vi "TMP007 Init.vi"(7 "I2C Channel":u8=1, 8 "error in (no error)":errorcluster, 9 "Samples to Average":u16(ring) items=["1 sample, .26s conversion"=0, "2 samples, .51s conversion"=512, "4 samples, 1.01s conversion"=1024, "8 samples, 2.01s conversion"=1536, "16 samples, 4.01s conversion"=2048], 10 "I2C Slave Address":u8=64 format="%.0x", 11 "LINX Resource in":T2) -> (0 "error out":errorcluster, 2 "Thermopile Setting":T1={"Samples to Average"=0, "I2C Slave Address"=64, "I2C Channel"=1, "Online"=FALSE} {"I2C Slave Address" format="%.0x"; "Samples to Average" items=["1 sample, .26s conversion"=0, "2 samples, .51s conversion"=512, "4 samples, 1.01s conversion"=1024, "8 samples, 2.01s conversion"=1536, "16 samples, 4.01s conversion"=2048]}, 3 "LINX Resource out":T2)   [LabVIEW 2014]
uses:
  <vilib>/MakerHub/LINX/Private/Type Defs/LINX Ref.ctl
  <vilib>/MakerHub/LINX/Private/Type Defs/Platform.ctl
  <vilib>/MakerHub/LINX/Private/Type Defs/Interface.ctl
  <vilib>/MakerHub/LINX/Private/Device/Type Defs/LINX Device Config.ctl
  <vilib>/MakerHub/LINX/Private/Device/Type Defs/TCP Config.ctl
  <vilib>/MakerHub/LINX/Private/Device/Type Defs/Channels.ctl
  <vilib>/MakerHub/LINX/Private/Local IO/LinxI2cWrite.vi
  <vilib>/MakerHub/LINX/Public/Utilities/Check Channel.vi
  <vilib>/myRIO/Instrument Drivers/Onboard IO/I2C/vis/Write.vi
  <vilib>/MakerHub/LINX/Private/Utilties/Generate Error.vi
  <vilib>/MakerHub/LINX/Private/Utilties/Channel FGVs/I2C Channels.vi
  <vilib>/Utility/error.llb/Error Cluster From Error Code.vi
  <vilib>/myRIO/Common/Instrument Driver Framework/myRIO v1.0/I2C/vis/myRIO v1.0 Write I2C.vi
  <vilib>/MakerHub/LINX/LMH-LINX.lvlib
  <vilib>/MakerHub/LINX/Private/Device/Device.lvlib
panel:
  # "Each sample takes .25s to convert\nThere are some other conversion modes that include idle times, but I didn't include those modes"
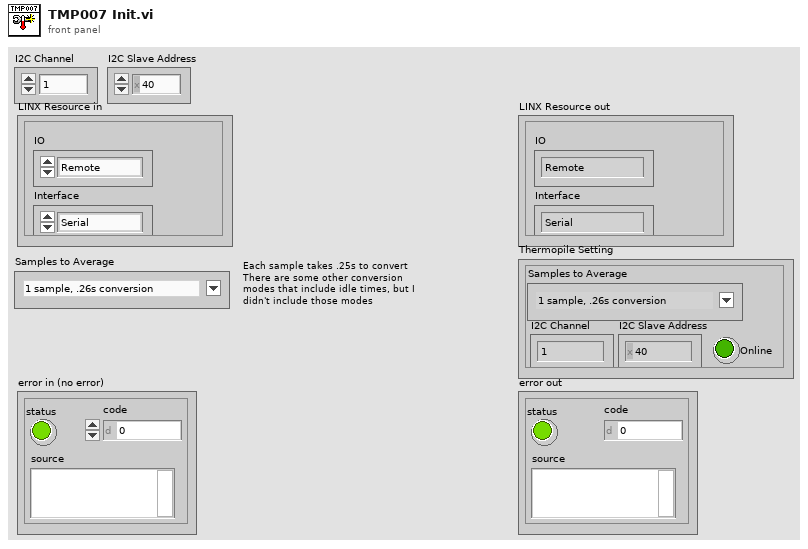
[diagram p1: front panel]
types:
  T1 = cluster{"Samples to Average":u16, "I2C Slave Address":u8, "I2C Channel":u8, "Online":bool}
  T2 = typedef "LMH-LINX.lvlib/LINX Ref.ctl" = cluster{"IO":T3, "Interface":T4, "LINX Device Config":T5}
  T3 = typedef "LMH-LINX.lvlib/Platform.ctl" = enum16{"Remote", "Local"}
  T4 = typedef "LMH-LINX.lvlib/Interface.ctl" = enum16{"Serial", "TCP"}
  T5 = typedef "LMH-LINX.lvlib/Device.lvlib/LINX Device Config.ctl" = cluster{"Interface":T4, "COM Port":refnum<visa-resource-name>, "TCP Configuration":T6, "Device Family":u8, "Device ID":u8, "Device Name":string, "TCP Ref":refnum<k5>, "Channels":T7}
  T6 = typedef "LMH-LINX.lvlib/Device.lvlib/TCP Config.ctl" = cluster{"IP Address":string, "Port":u16}
  T7 = typedef "LMH-LINX.lvlib/Channels.ctl" = cluster{"DI":u8[], "DO":u8[], "AI":u8[], "AO":u8[], "PWM":u8[], "QE":u8[], "UART":u8[], "I2C 2":u8[], "SPI":u8[], "CAN":u8[], "Servo":u8[], "AI Ref (V)":dbl, "AI Resolution (Bits)":u8, "AO Ref (V)":dbl, "AO Resolution (Bits)":u8}
  T8 = cluster{"Samples to Average":u16, "I2C Slave Address":u8, "I2C Channel":u8, bool}
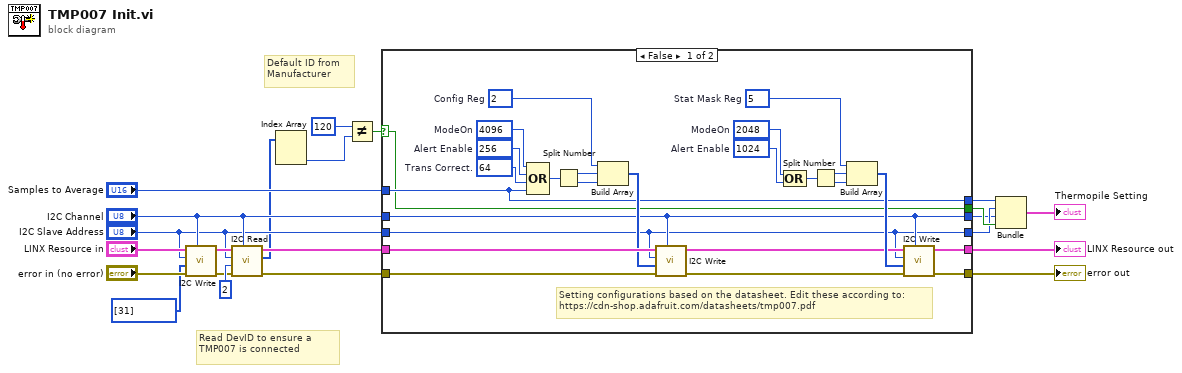
[diagram p0: block diagram]
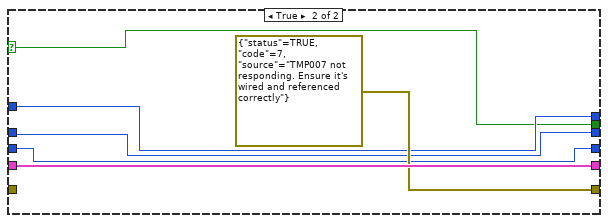
[diagram p2: hidden frame]
diagram:
  # "Default ID from Manufacturer"
  # "Read DevID to ensure a TMP007 is connected"
  n1 = call <vilib>:"I2C Write.vi"("I2C Channel"="I2C Channel", "Error In"="error in (no error)", "Data"=u8[] [31], "I2C Slave Address (0)"="I2C Slave Address", "LINX Resource"="LINX Resource in") -> ("Error Out"=w15:errorcluster, "LINX Resource"=w14:T2)  [unwired: 5 in]
  n2 = call <vilib>:"I2C Read.vi"("I2C Channel"="I2C Channel", "Error In"=w15, "Bytes To Read"=u8 2, "I2C Slave Address (0)"="I2C Slave Address", "LINX Resource"=w14) -> ("Error Out"=w18:errorcluster, "Data"=w8:u8[], "LINX Resource"=w19:T2)  [unwired: 4 in]
  n3 = Index Array(array=w8) -> (element #2=w6:u8)  [unwired: 2 in, 1 out]
  n4 = Not Equal?(x=u8 120, y=w6) -> (x != y?=w12:bool)
  n5 = case shown="False" w12 {
    selector: w12 -> [w25 w50]
    tunnel: w19 -> [w47 w53]
    tunnel: [w28 w53] -> w21
    tunnel: w18 -> [w46 _]
    tunnel: [w27 errorcluster {"status"=TRUE, "code"=7, "source"="TMP007 not responding. Ensure it's wired and referenced correctly"} ("error constant")] -> w20
    tunnel: "Samples to Average" -> [w26 w51]
    tunnel: "I2C Channel" -> [w24 w49]
    tunnel: "I2C Slave Address" -> [w23 w48]
    tunnel: [w26 w51] -> w5
    tunnel: [w25 w50] -> w4
    tunnel: [w24 w49] -> w1
    tunnel: [w23 w48] -> w2
    frame False {
      w37 = u8 5  # Stat Mask Reg
      w32 = u16 1024  # Alert Enable
      w33 = u16 2048  # ModeOn
      w39 = u8 2  # Config Reg
      w45 = u16 64  # Trans Correct.
      w44 = u16 256  # Alert Enable
      w43 = u16 4096  # ModeOn
      # "Setting configurations based on the datasheet. Edit these according to:\nhttps://cdn-shop.adafruit.com/datasheets/tmp007.pdf"
      n6 = Compound Arithmetic op=OR(w43, w44, w45, w26) -> (w42:u16)
      n7 = Split Number(x=w42) -> (hi(x)=w41:u8, lo(x)=w40:u8)
      n8 = Build Array(w39, w41, w40) -> (w38:u8[])
      n9 = call <vilib>:"I2C Write.vi"("I2C Channel"=w24, "Error In"=w46, "Data"=w38, "I2C Slave Address (0)"=w23, "LINX Resource"=w47) -> ("Error Out"=w29:errorcluster, "LINX Resource"=w30:T2)  [unwired: 5 in]
      n10 = Compound Arithmetic op=OR(w33, w32) -> (w34:u16)
      n11 = Split Number(x=w34) -> (hi(x)=w35:u8, lo(x)=w36:u8)
      n12 = Build Array(w37, w35, w36) -> (w31:u8[])
      n13 = call <vilib>:"I2C Write.vi"("I2C Channel"=w24, "Error In"=w29, "Data"=w31, "I2C Slave Address (0)"=w23, "LINX Resource"=w30) -> ("Error Out"=w27:errorcluster, "LINX Resource"=w28:T2)  [unwired: 5 in]
    }
    frame True {
    }
  }
  "error out" <- w20
  "LINX Resource out" <- w21
  n14 = Bundle("Samples to Average"=w5, "I2C Slave Address"=w2, "I2C Channel"=w1, w4) -> (→"Thermopile Setting":T8)  [unwired: 1 in]
